vi "packData2string_multiAxis.vi"(9 "F_i: current freq":dbl, 10 "output cluster":cluster{"z-err data":dbl[], "u_z-data":dbl[]}) -> (2 "spreadsheet string":string)   [LabVIEW 2017]
doc: "This VI takes the acquired data stream, pre-pends the current frequency and total number of elements in the array. Then, it converts the array of doubles into a spreadsheet string, with format,\n\n'%f, %f, ...'"
panel:
  out "appended array":dbl[][](array[numeric])
  # "f_i         axisID  data     dat1   dat2   ....                                        datn\n                        len =n"
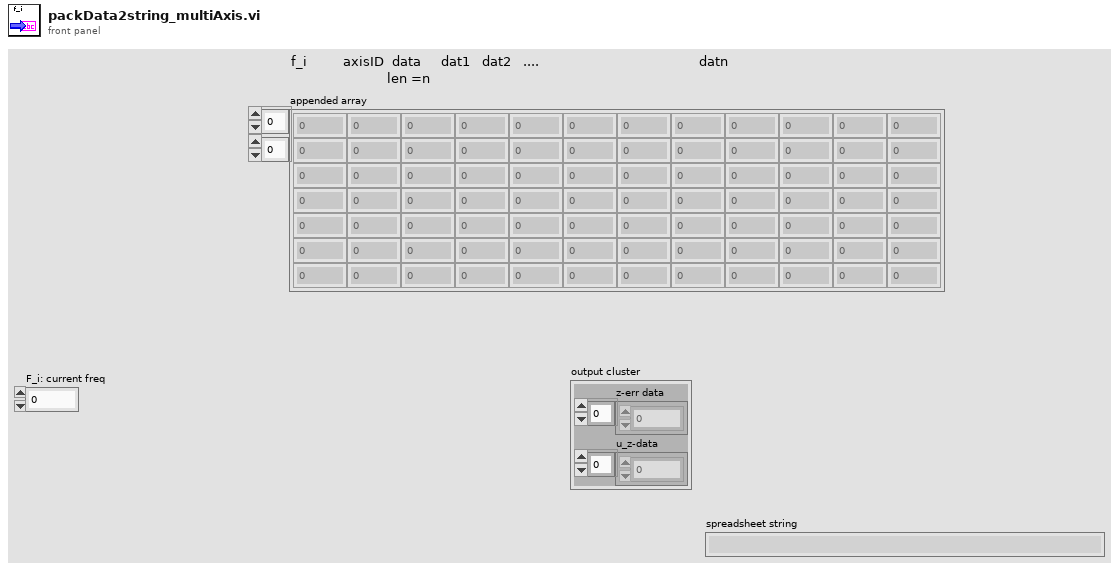
[diagram p1: front panel]
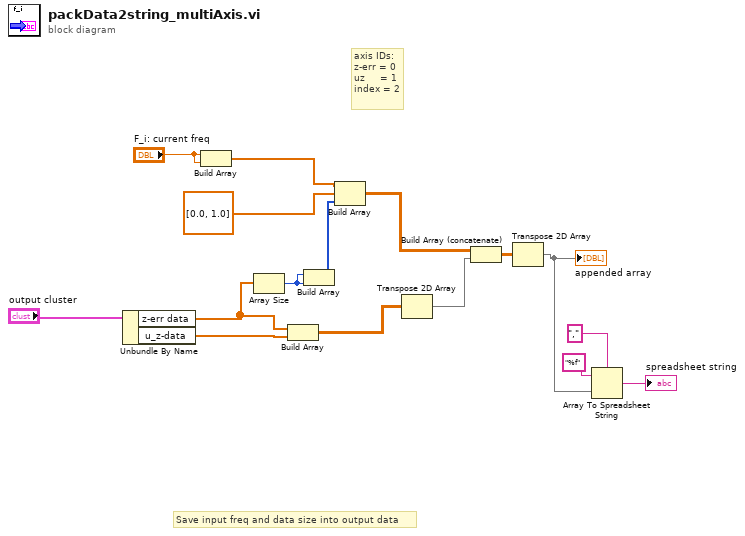
[diagram p0: block diagram]
diagram:
  # "axis IDs:\nz-err = 0\nuz     = 1\nindex = 2"
  # "Save input freq and data size into output data"
  n1 = Unbundle By Name("output cluster") -> ("z-err data"=w12:dbl[], "u_z-data"=w15:dbl[])
  n2 = Build Array("F_i: current freq", "F_i: current freq") -> (w14:dbl[])
  n3 = Array Size(array=w12) -> (size(s)=w11:i32)
  n4 = Build Array(w12, w15) -> (w9:dbl[][])
  n5 = Build Array(w11, w11) -> (w10:i32[])
  n6 = Build Array(w14, sgl[] [0.0, 1.0], w10) -> (w8:dbl[][])
  n7 = Transpose 2D Array(2D array=w9) -> (transposed array=w7:dbl[][])
  n8 = Build Array (concatenate)(w8, w7) -> (w6:dbl[][])
  n9 = Transpose 2D Array(2D array=w6) -> (transposed array=w3:dbl[][])
  "appended array" <- w3
  n10 = Array To Spreadsheet String(delimiter (Tab)=",", array=w3, 3:"%f") -> (spreadsheet string=→"spreadsheet string":string)
